vi "Teleop Shooter Control.vi"(9 "D-Pad":T1, 10 "Manipulator Button Cluster":T3, 11 "Manipulator Axes Cluster":T2) -> ()   [LabVIEW 2016]
uses:
  Common Code/Gamepads/Button Cluster.ctl
  Common Code/Gamepads/Axes Cluster.ctl
  Common Code/Gamepads/D-Pad.ctl
  Common Code/Shooter Modes.ctl
  Common Code/Shot Type.ctl
  Common Code/Shooter Commands.ctl
  Common Code/Utilities/Change Detect.vi
  Common Code/Utilities/Change Detect Boolean.vi
  Robot Global Data.vi
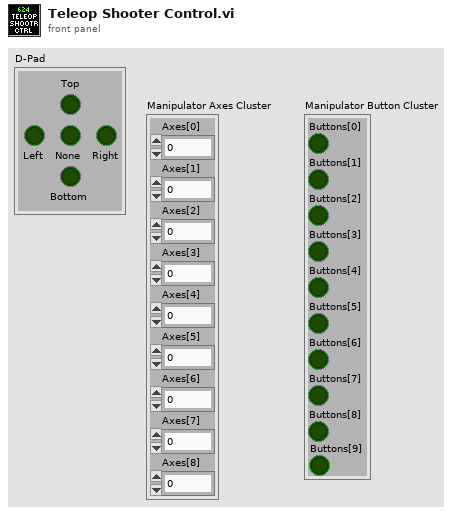
[diagram p1: front panel]
types:
  T1 = typedef "D-Pad.ctl" = cluster{"Top":bool, "Bottom":bool, "None":bool, "Right":bool, "Left":bool}
  T2 = typedef "Axes Cluster.ctl" = cluster{"Axes[0]":dbl, "Axes[1]":dbl, "Axes[2]":dbl, "Axes[3]":dbl, "Axes[4]":dbl, "Axes[5]":dbl, "Axes[6]":dbl, "Axes[7]":dbl, "Axes[8]":dbl}
  T3 = typedef "Button Cluster.ctl" = cluster{"Buttons[0]":bool, "Buttons[1]":bool, "Buttons[2]":bool, "Buttons[3]":bool, "Buttons[4]":bool, "Buttons[5]":bool, "Buttons[6]":bool, "Buttons[7]":bool, "Buttons[8]":bool, "Buttons[9]":bool}
  T4 = enum16{"0", "1", "2", "3", "4", "5", "6", "7", "8", "9", "A", "B", "C", "D", "E", "F", "G", "H", "I", "J", "K", "L", "M", "N", "O", "P", "Q", "R", "S", "T", "U", "V", "W", "X", "Y", "Z", "F1", "F2", "F3", "F4", "F5", "F6", "F7", "F8", "F9", "F10", "F11", "F12", "F13", "F14", "F15", "ADD", "BACK", "BACKSLASH", "CAPITAL", "COMMA", "DECIMAL", "DELETE", "DIVIDE", "DOWN", "END", "EQUALS", "ESCAPE", "GRAVE (`)", "HOME", "INSERT", "LBRACKET", "LCONTROL", "LEFT", "L ALT", "LSHIFT", "LWIN", "MINUS", "MULTIPLY", "NEXT", "NUMLOCK", "NUMPAD_0", "NUMPAD_1", "NUMPAD_2", "NUMPAD_3", "NUMPAD_4", "NUMPAD_5", "NUMPAD_6", "NUMPAD_7", "NUMPAD_8", "NUMPAD_9", "PAUSE", "PERIOD", "PRIOR (PG UP)", "RBRACKET", "RCONTROL", "RETURN", "RIGHT", "R ALT", "RSHIFT", "RWIN", "SCROLL", "SEMICOLON", "SLASH", "SPACE", "SUBTRACT", "TAB", "UP", "ENTER (num pad)", "' (quote)"}
  T5 = typedef "Shooter Commands.ctl" = enum16{"Idle ", "Warmup ", "Shoot"}
  T6 = typedef "Shot Type.ctl" = enum16{"Vision Shot", "Dist Shot", "Key Shot"}
  T7 = typedef "Shooter Modes.ctl" = enum16{"Auto", "Manual"}
  T8 = typedef "Shooter Control Cluster'.ctl" = cluster{"Shooter Modes":T7, "Shooter Commands":T5, "manUEL Control Cluster":T9, "Shot Type":T6}
  T9 = typedef "Manual Shoot Cluster.ctl" = cluster{"Shot RPM":dbl, "Wait Time":dbl, "da HOOD?":bool}
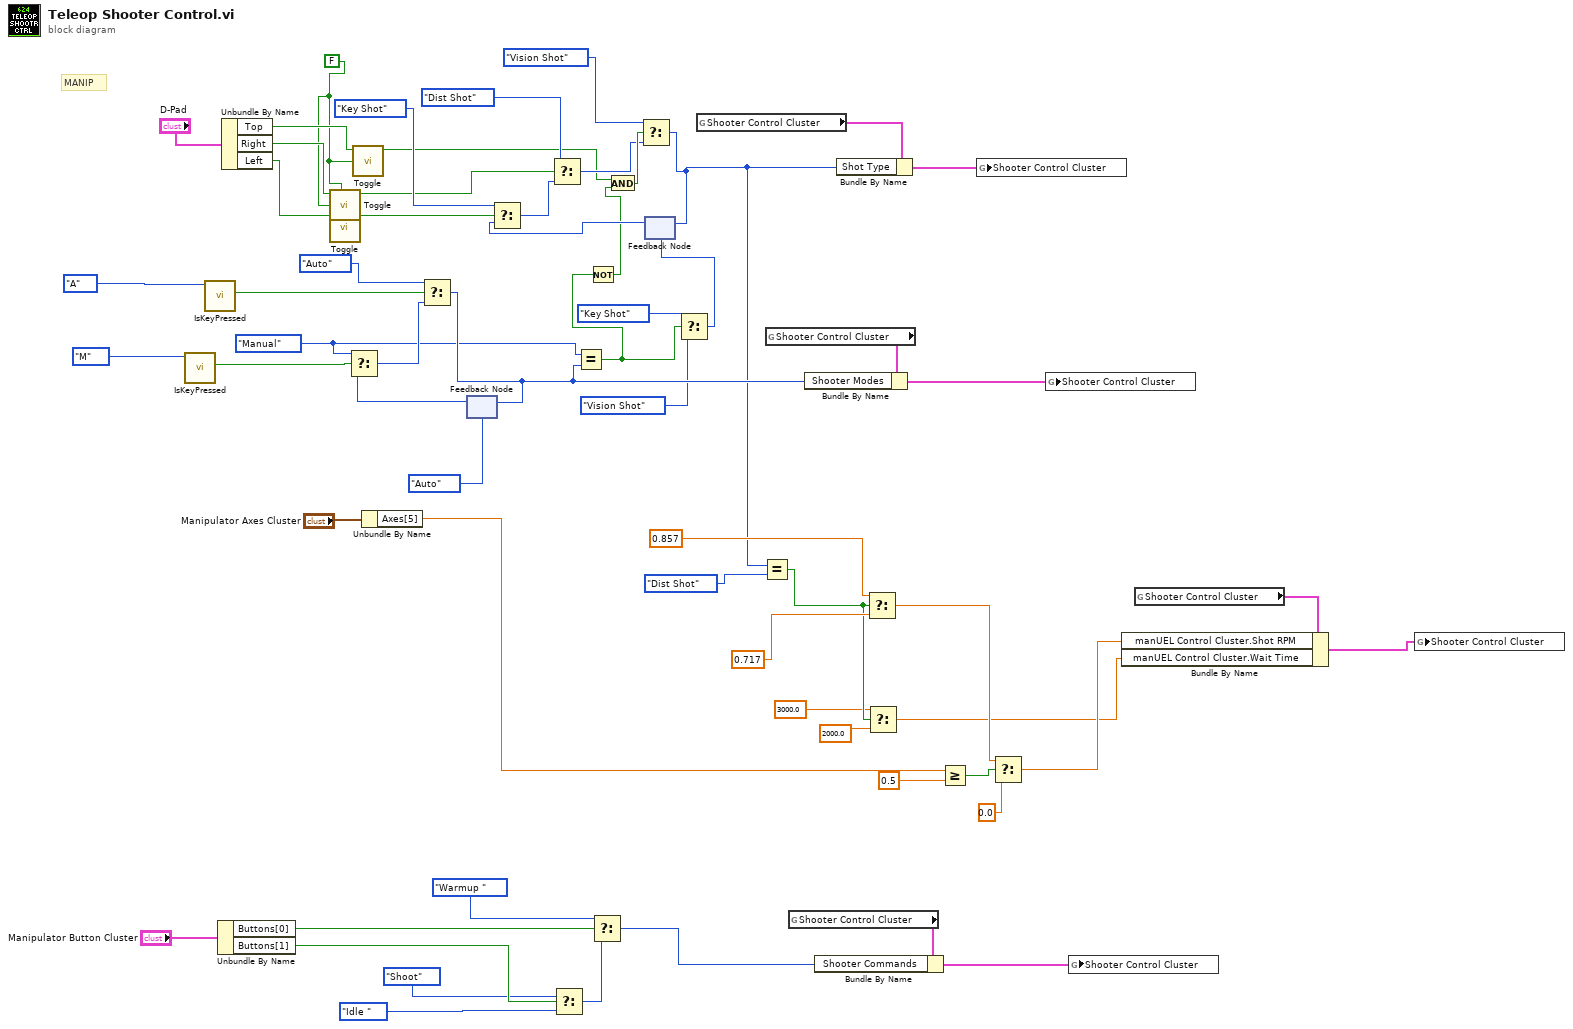
[diagram p0: block diagram]
diagram:
  w1 = FALSE
  w39 = Shooter_Modes."Manual" ("Shooter Modes")
  # "MANIP"
  n1 = call "IsKeyPressed.vi"("Key Pressed"=T4."M" ("keyType 3")) -> ("Key Down?"=w51:bool)  [unwired: 10 in]
  n2 = call "IsKeyPressed.vi"("Key Pressed"=T4."A" ("keyType 3")) -> ("Key Down?"=w54:bool)  [unwired: 10 in]
  n3 = Unbundle By Name("Manipulator Button Cluster") -> ("Buttons[0]"=w9:bool, "Buttons[1]"=w13:bool)
  n4 = Unbundle By Name("D-Pad") -> ("Top"=w21:bool, "Right"=w19:bool, "Left"=w17:bool)
  n5 = call "Toggle.vi"("Initial Value"=w1, "In"=w19) -> ("Toggled"=w18:bool)  [unwired: 9 in]
  n6 = call "Toggle.vi"("Initial Value"=w1, "In"=w17) -> ("Toggled"=w16:bool)  [unwired: 9 in]
  n7 = call "Toggle.vi"("Initial Value"=w1, "In"=w21) -> ("Toggled"=w20:bool)  [unwired: 9 in]
  n8 = Unbundle By Name("Manipulator Axes Cluster") -> ("Axes[5]"=w58:dbl)
  n9 = feedback #1(Shooter_Modes."Auto" ("Shooter Modes")) -> (w49:T7)
  n10 = Select(t=w39, s=w51, f=w49) -> (s? t:f=w52:T7)
  n11 = Select(t=Shooter_Modes."Auto" ("Shooter Modes"), s=w54, f=w52) -> (s? t:f=w40:T7)
  n12 = feedback-in #1(w40) -> ()
  n13 = Select(t=Shooter_Commands."Shoot" ("Shooter Commands"), s=w13, f=Shooter_Commands."Idle " ("Shooter Commands")) -> (s? t:f=w12:T5)
  n14 = Equal?(x=w39, y=w40) -> (x = y?=w35:bool)
  n15 = Not(x=w35) -> (.not. x?=w34:bool)
  n16 = Select(t=Shooter_Commands."Warmup " ("Shooter Commands"), s=w9, f=w12) -> (s? t:f=w8:T5)
  n17 = And(x=w20, y=w34) -> (x .and. y?=w33:bool)
  n18 = Select(t=Shot_Type."Key Shot" ("Shot Type"), s=w35, f=Shot_Type."Vision Shot" ("Shot Type")) -> (s? t:f=w36:T6)
  n19 = feedback #2(w36) -> (w41:T6)
  n20 = Select(t=Shot_Type."Key Shot" ("Shot Type"), s=w16, f=w41) -> (s? t:f=w43:T6)
  n21 = Select(t=Shot_Type."Dist Shot" ("Shot Type"), s=w18, f=w43) -> (s? t:f=w32:T6)
  n22 = Select(t=Shot_Type."Vision Shot" ("Shot Type"), s=w33, f=w32) -> (s? t:f=w15:T6)
  n23 = feedback-in #2(w15) -> ()
  n24 = global read "Robot Global Data.vi" "Shooter Control Cluster"() -> (w48:T8)
  n25 = Equal?(x=w15, y=Shot_Type."Dist Shot" ("Shot Type")) -> (x = y?=w7:bool)
  n26 = global read "Robot Global Data.vi" "Shooter Control Cluster"() -> (w55:T8)
  n27 = global read "Robot Global Data.vi" "Shooter Control Cluster"() -> (w23:T8)
  n28 = Bundle By Name(cluster=w55, "Shooter Modes"=w40) -> (w56:T8)
  n29 = Bundle By Name(cluster=w23, "Shooter Commands"=w8) -> (w22:T8)
  n30 = Bundle By Name(cluster=w48, "Shot Type"=w15) -> (w47:T8)
  n31 = Select(t=0.857, s=w7, f=0.717) -> (s? t:f=w27:dbl)
  n32 = Select(t=3000.0, s=w7, f=2000.0) -> (s? t:f=w4:dbl)
  n33 = Greater Or Equal?(x=w58, y=0.5) -> (x >= y?=w28:bool)
  n34 = global write "Robot Global Data.vi" "Shooter Control Cluster"(w47) -> ()
  n35 = Select(t=w27, s=w28, f=0.0) -> (s? t:f=w25:dbl)
  n36 = global write "Robot Global Data.vi" "Shooter Control Cluster"(w56) -> ()
  n37 = global write "Robot Global Data.vi" "Shooter Control Cluster"(w22) -> ()
  n38 = global read "Robot Global Data.vi" "Shooter Control Cluster"() -> (w60:T8)
  n39 = Bundle By Name(cluster=w60, "manUEL Control Cluster.Shot RPM"=w25, "manUEL Control Cluster.Wait Time"=w4) -> (w59:T8)
  n40 = global write "Robot Global Data.vi" "Shooter Control Cluster"(w59) -> ()
